vi "Test Get Controls Indicators.vi"() -> ()   [LabVIEW 2014]
panel:
  out "Data Type":string[](array[string])
  out "error in label":string
  out "error out label":string
  out "#indicators":i32
  out "#controls":i32
  in  "DataType":string(combo)="error"
  in  "vi path":path=path "C:/Users/lubo/Documents/LabView/LabVIEW-Universal-Transcriptor/Test/Example Test 1.vi"
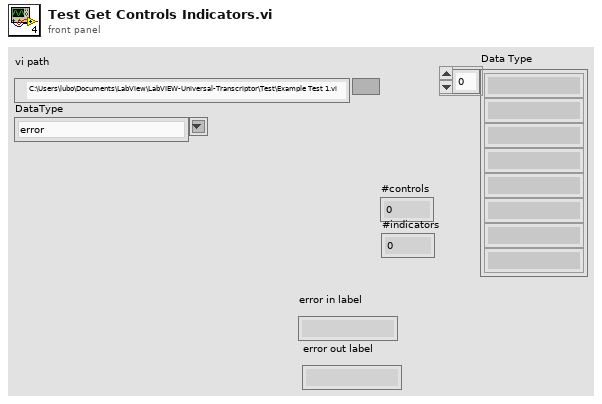
[diagram p1: front panel]
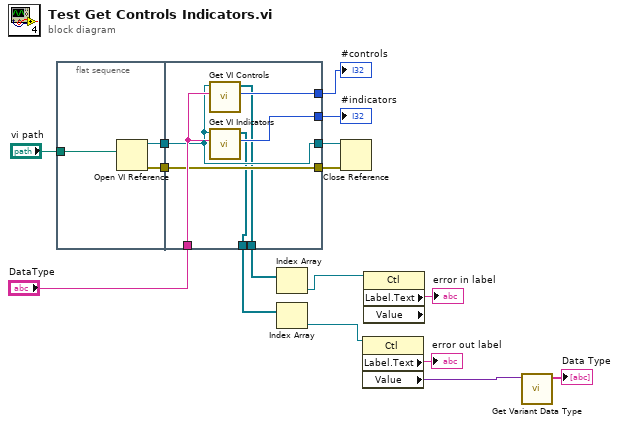
[diagram p0: block diagram]
diagram:
  n1 = flat-sequence {
    tunnel: "vi path" -> [w19]
    tunnel: [w18] -> w15
    tunnel: [w17] -> w10
    tunnel: w15 -> [w22]
    tunnel: "DataType" -> [w26]
    tunnel: [w25] -> w13
    tunnel: [w24] -> w12
    tunnel: [w23] -> w11
    tunnel: w10 -> [w23]
    tunnel: [w22] -> w9
    tunnel: [w21] -> w8
    tunnel: [w20] -> w7
    frame #0 {
      n2 = Open VI Reference(vi path=w19) -> (vi reference=w18:refnum<vi>, error out=w17:errorcluster)  [unwired: 5 in]
    }
    frame #1 {
      n3 = call "Get VI Controls.vi"("DataType"=w26, "VI ref."=w22) -> ("#controls"=w25:i32, "Controls Array"=w21:refnum<vi>[])  [unwired: 8 in]
      n4 = call "Get VI Indicators.vi"("DataType"=w26, "VI ref."=w22) -> ("#indicators"=w24:i32, "Controls Array"=w20:refnum<vi>[])  [unwired: 8 in]
    }
  }
  n5 = Index Array(array=w8) -> (element=w6:refnum<vi>)  [unwired: 1 in]
  n6 = Index Array(array=w7) -> (element=w5:refnum<vi>)  [unwired: 1 in]
  n7 = Close Reference(reference=w9, error in (no error)=w11) -> ()  [unwired: 1 out]
  n8 = property class="Ctl"(reference=w5) -> ("Label.Text"=→"error out label":string, "Value"=w1:variant)  [unwired: 1 in, 2 out]
  n9 = property class="Ctl" props=["Label", "Text", "Value"](reference=w6) -> ("Label.Text"=→"error in label":string)  [unwired: 1 in, 3 out]
  n10 = call "Get Variant Data Type.vi"("Variant in"=w1) -> ("Data Types[]"=→"Data Type":string[])  [unwired: 9 in, 1 out]
  "#controls" <- w13
  "#indicators" <- w12
